vi "Image Display And Save 2.vi"() -> ()   [LabVIEW 2018]
doc: "Image Display And Save2: This example is an example of image reading, display, and saving. It uses the mat_to_2d_pic.vi function to display an image and the imwrite.vi function to save the image to a file."
uses:
  vi.lib/VIRobotics/opencv_yiku/ctls/ColorConversionCodes.ctl
  vi.lib/VIRobotics/opencv_yiku/Mat/Mat_8U/Mat_8U.lvclass
  D:/Program Files/company/National Instruments/LabVIEW 2018/vi.lib/addons/VIRobotics/opencv_yiku/Mat/Mat/Mat.lvclass
  vi.lib/VIRobotics/opencv_yiku/Mat/Create_Mat_8U.vi
  vi.lib/VIRobotics/opencv_yiku/Mat/Mat/Mat_release.vi
  vi.lib/VIRobotics/opencv_yiku/opencv_yiku.lvlib
  vi.lib/VIRobotics/opencv_yiku/Mat/Mat/Mat.lvclass
panel:
  out "src out":picture
  out "dst out":picture
  # "Overview: Demonstrates how to load an image, display it in a picture control, and save it to a file.\nRequirements: Windows.\nInstructions: \n1. Run the VI."
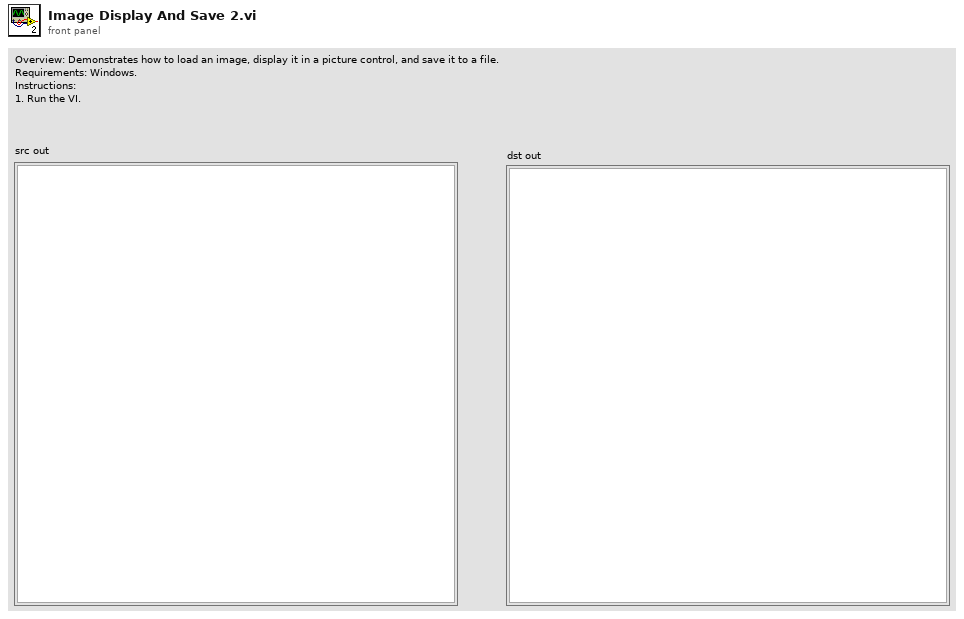
[diagram p1: front panel]
types:
  T1 = typedef "opencv_yiku.lvlib/ColorConversionCodes.ctl" = enum32{"COLOR_BGR2BGRA", "COLOR_BGRA2BGR", "COLOR_BGR2RGBA", "COLOR_RGBA2BGR", "COLOR_BGR2RGB", "COLOR_BGRA2RGBA", "COLOR_BGR2GRAY", "COLOR_RGB2GRAY", "COLOR_GRAY2BGR", "COLOR_GRAY2BGRA", "COLOR_BGRA2GRAY", "COLOR_RGBA2GRAY", "COLOR_BGR2BGR565", "COLOR_RGB2BGR565", "COLOR_BGR5652BGR", "COLOR_BGR5652RGB", "COLOR_BGRA2BGR565", "COLOR_RGBA2BGR565", "COLOR_BGR5652BGRA", "COLOR_BGR5652RGBA", "COLOR_GRAY2BGR565", "COLOR_BGR5652GRAY", "COLOR_BGR2BGR555", "COLOR_RGB2BGR555", "COLOR_BGR5552BGR", "COLOR_BGR5552RGB", "COLOR_BGRA2BGR555", "COLOR_RGBA2BGR555", "COLOR_BGR5552BGRA", "COLOR_BGR5552RGBA", "COLOR_GRAY2BGR555", "COLOR_BGR5552GRAY", "COLOR_BGR2XYZ", "COLOR_RGB2XYZ", "COLOR_XYZ2BGR", "COLOR_XYZ2RGB", "COLOR_BGR2YCrCb", "COLOR_RGB2YCrCb", "COLOR_YCrCb2BGR", "COLOR_YCrCb2RGB", "COLOR_BGR2HSV", "COLOR_RGB2HSV", "42", "43", "COLOR_BGR2Lab", "COLOR_RGB2Lab"}
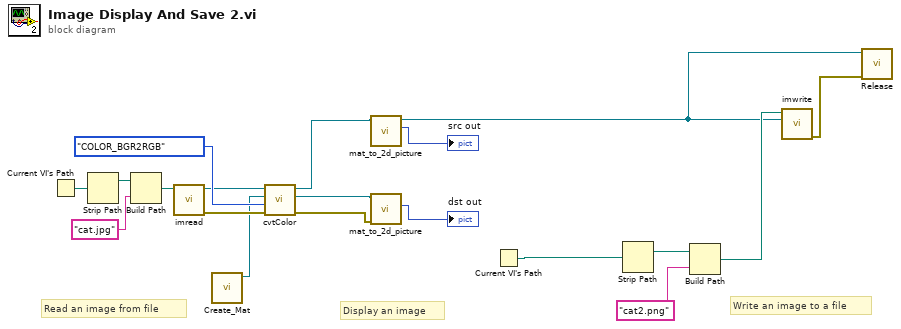
[diagram p0: block diagram]
diagram:
  # "Write an image to a file"
  # "Display an image"
  # "Read an image from file"
  n1 = Current VI's Path() -> (path=w19:path)
  n2 = Strip Path(path=w19) -> (stripped path=w18:path)  [unwired: 1 out]
  n3 = Build Path(base path=w18, name or relative path="cat.jpg") -> (appended path=w16:path)
  n4 = call "imread.vi"("path"=w16) -> ("error out"=w14:errorcluster, "Mat out"=w13:refnum<class "Mat_8U.lvclass">)  [unwired: 9 in]
  n5 = call-poly "Create_Mat.vi"() -> ("Mat_8U_out"=w12:refnum<class "Mat_8U.lvclass">)  [unwired: 10 in, 1 out]
  n6 = call "cvtColor.vi"("error in (no error)"=w14, "dstCn"=ColorConversionCodes."COLOR_BGR2RGB", "dst"=w12, "src"=w13) -> ("error out"=w4:errorcluster, "dst out"=w5:refnum<class "Mat_8U.lvclass">, "src out"=w7:refnum<class "Mat_8U.lvclass">)  [unwired: 5 in]
  n7 = call "mat_to_2d_picture.vi"("Mat_8U in"=w7) -> ("picture"=→"src out":picture, "Mat_8U out"=w2:refnum<class "Mat_8U.lvclass">)  [unwired: 8 in, 1 out]
  n8 = call "mat_to_2d_picture.vi"("error in (no error)"=w4, "Mat_8U in"=w5) -> ("picture"=→"dst out":picture)  [unwired: 7 in, 2 out]
  n9 = Current VI's Path() -> (path=w11:path)
  n10 = Strip Path(path=w11) -> (stripped path=w10:path)  [unwired: 1 out]
  n11 = Build Path(base path=w10, name or relative path="cat2.png") -> (appended path=w8:path)
  n12 = call "imwrite.vi"("Mat out"=w2, "path"=w8) -> ("error out"=w1:errorcluster)  [unwired: 9 in]
  n13 = call-poly "Release.vi"("error in (no error)"=w1, "Mat in"=w2) -> ()  [unwired: 9 in, 1 out]
